vi "Set Just Validate.vi"(8 "error in (no error)":errorcluster, 10 "Just Validate":bool, 11 "CFG JSON Base in":refnum<class "CFG JSON Base.lvclass">) -> (0 "error out":errorcluster, 3 "CFG JSON Base out":refnum<class "CFG JSON Base.lvclass">)   [LabVIEW 2023, in "HAL GOOP4.lvlib" / "CFG JSON Base.lvclass"]
uses:
  CFG JSON Base.lvclass
  CFG JSON Base.lvclass/CFG JSON Base.ctl
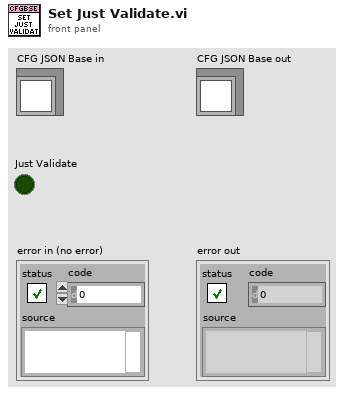
[diagram p1: front panel]
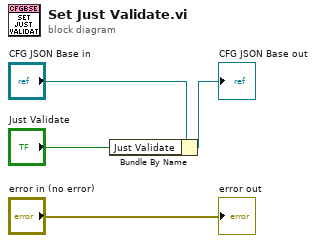
[diagram p0: block diagram]
diagram:
  n1 = Bundle By Name(cluster="CFG JSON Base in", "Just Validate"="Just Validate") -> (→"CFG JSON Base out":refnum<class "CFG JSON Base.lvclass">)
  "error out" <- "error in (no error)"
